vi "字符串比对X.vi"(11 "字符串":string) -> (3 "布尔":bool)   [LabVIEW 2021]
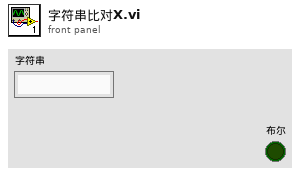
[diagram p1: front panel]
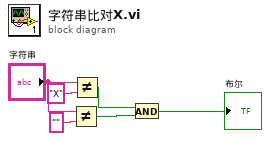
[diagram p0: block diagram]
diagram:
  n1 = Not Equal?(x="字符串", y="") -> (x != y?=w2:bool)
  n2 = Not Equal?(x="字符串", y="X") -> (x != y?=w3:bool)
  n3 = And(x=w3, y=w2) -> (x .and. y?=→"布尔":bool)
